vi "Balloon.vi"(1 "One more?":bool, 2 "Latitude":dbl format="%#.6g", 3 "character":string, 4 "color":string(combo), 6 "Longitude":dbl format="%#.6g") -> (0 "Balloon":string)   [LabVIEW 2015]
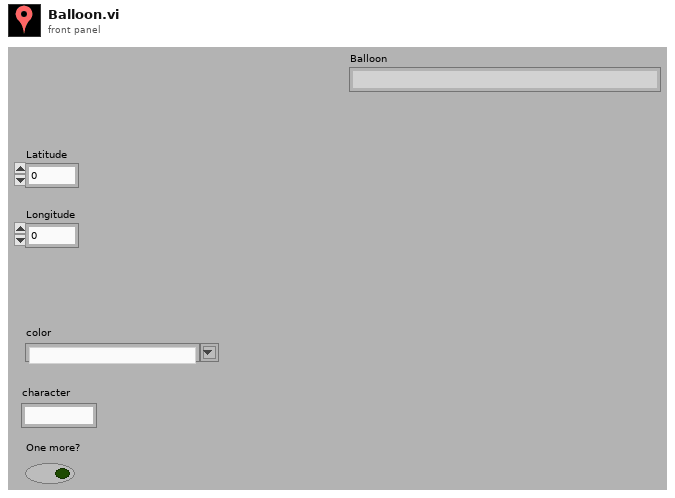
[diagram p1: front panel]
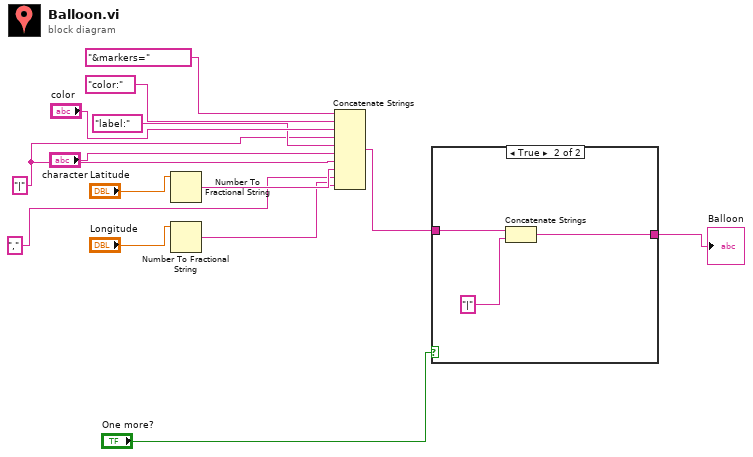
[diagram p0: block diagram]
diagram:
  w4 = "|"
  n1 = Number To Fractional String(number="Latitude") -> (F-format string=w3:string)  [unwired: 3 in]
  n2 = Number To Fractional String(number="Longitude") -> (F-format string=w1:string)  [unwired: 3 in]
  n3 = Concatenate Strings("&markers=", "color:", "color", w4, "label:", "character", w4, w3, ",", w1) -> (w11:string)
  n4 = case shown="True" "One more?" {
    tunnel: w11 -> [w15 w18]
    tunnel: [w15 w16] -> w10
    frame False {
    }
    frame True {
      n5 = Concatenate Strings(w18, "|") -> (w16:string)
    }
  }
  "Balloon" <- w10
